vi "send stop.vi"(8 "error in (no error)":errorcluster, 11 "port (5555)":i32=5555) -> (0 "error out":errorcluster)   [LabVIEW 2020, in "splash_screen.lvlib"]
uses:
  splash_screen.lvlib
  <vilib>/addons/zeromq/socket_type.ctl
  <vilib>/addons/zeromq/zmq_context.lvclass
  <vilib>/addons/zeromq/zeromq.lvlib
  <vilib>/addons/zeromq/zmq_socket.lvclass
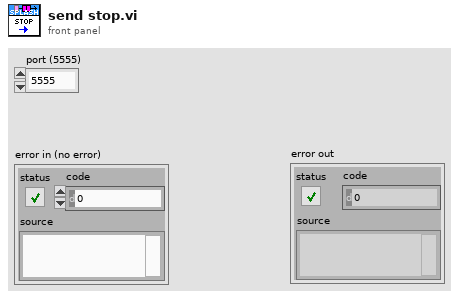
[diagram p1: front panel]
types:
  T1 = typedef "zeromq.lvlib/socket_type.ctl" = enum8{"ZMQ_PAIR", "ZMQ_PUB", "ZMQ_SUB", "ZMQ_REQ", "ZMQ_REP", "ZMQ_DEALER", "ZMQ_ROUTER", "ZMQ_PULL", "ZMQ_PUSH", "ZMQ_XPUB", "ZMQ_XSUB", "ZMQ_STREAM", "ZMQ_SERVER", "ZMQ_CLIENT", "ZMQ_RADIO", "ZMQ_DISH", "ZMQ_GATHER", "ZMQ_SCATTER", "ZMQ_DGRAM"}
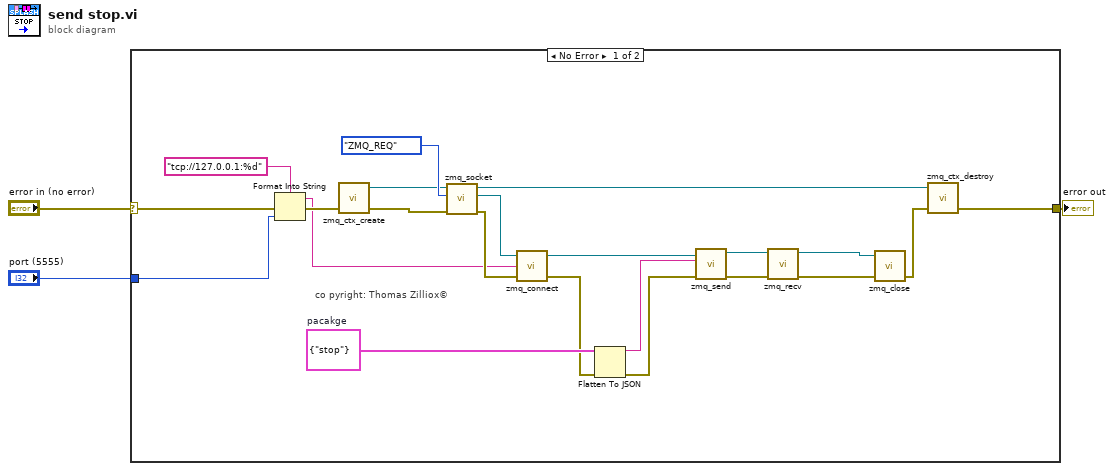
[diagram p0: block diagram]
diagram:
  n1 = case shown="No Error" "error in (no error)" {
    selector: "error in (no error)" -> [w17 w26]
    tunnel: [w13 w26] -> w2
    tunnel: "port (5555)" -> [w16 _]
    frame No Error {
      w8 = cluster{"message":string} {"message"="stop"}  # pacakge
      # "co pyright: Thomas Zilliox©"
      n2 = Format Into String(format string="tcp://127.0.0.1:%d", error in=w17, w16) -> (resulting string=w4:string, error out=w14:errorcluster)  [unwired: 1 in]
      n3 = call <vilib>:"zmq_ctx_create.vi"("error in"=w14) -> ("error out"=w19:errorcluster, "context out"=w18:refnum<class "zmq_context.lvclass">)  [unwired: 3 in]
      n4 = call <vilib>:"zmq_socket.vi"("error in"=w19, "socket type"=socket_type."ZMQ_REQ", "context in"=w18) -> ("error out"=w23:errorcluster, "socket out"=w22:refnum<class "zmq_socket.lvclass">, "context out"=w21:refnum<class "zmq_context.lvclass">)  [unwired: 2 in]
      n5 = call <vilib>:"zmq_connect.vi"("error in"=w23, "endpoint"=w4, "socket in"=w22) -> ("error out"=w7:errorcluster, "socket out"=w24:refnum<class "zmq_socket.lvclass">)  [unwired: 1 in]
      n6 = Flatten To JSON(anything=w8, error in (no error)=w7) -> (JSON string=w5:string, 11:w6:errorcluster)  [unwired: 1 in]
      n7 = call <vilib>:"zmq_send.vi"("error in"=w6, "data"=w5, "socket in"=w24) -> ("error out"=w11:errorcluster, "socket out"=w12:refnum<class "zmq_socket.lvclass">)  [unwired: 4 in]
      n8 = call <vilib>:"zmq_recv.vi"("error in"=w11, "socket in"=w12) -> ("error out"=w10:errorcluster, "socket out"=w9:refnum<class "zmq_socket.lvclass">)  [unwired: 3 in, 3 out]
      n9 = call <vilib>:"zmq_close.vi"("error in"=w10, "socket"=w9) -> ("error out"=w25:errorcluster)  [unwired: 3 in]
      n10 = call <vilib>:"zmq_ctx_destroy.vi"("error in"=w25, "context in"=w21) -> ("error out"=w13:errorcluster)  [unwired: 3 in]
    }
    frame Error {
    }
  }
  "error out" <- w2
